vi "Init.vi"(8 "error in (no error)":errorcluster, 11 "reference in":refnum<class "TestView_Base.lvclass">) -> (0 "error out":errorcluster, 3 "reference in":refnum<class "TestView_Base.lvclass">)   [LabVIEW 2022 SP3, in "TestView_Base.lvlib" / "TestView_Base.lvclass"]
uses:
  TestView_Base.lvclass
  Components/ViPER.lvlibp/ViPER.lvclass
  C:/Projects/Medulla/ViPER/Examples/Flux_Capacitor_Tester/Components/ViPER.lvlibp/ViPER.lvclass
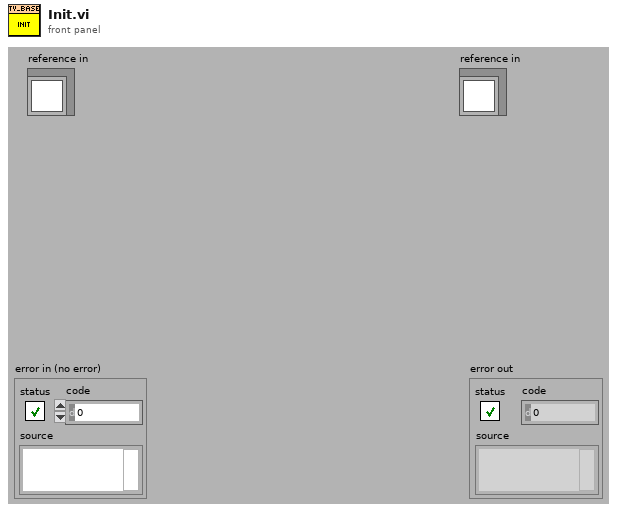
[diagram p1: front panel]
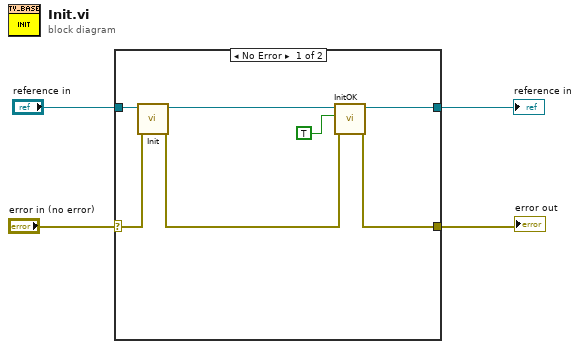
[diagram p0: block diagram]
diagram:
  n1 = case shown="No Error" "error in (no error)" {
    selector: "error in (no error)" -> [w10 w13]
    tunnel: [w8 w13] -> w3
    tunnel: [w9 w12] -> w1
    tunnel: "reference in" -> [w11 w12]
    frame No Error {
      n2 = call-parent "Init.vi"("error in (no error)"=w10, "reference in"=w11) -> ("error out"=w5:errorcluster, "reference out"=w6:refnum<class "TestView_Base.lvclass">)  [unwired: 8 in]
      n3 = call "InitOK.vi"("error in (no error)"=w5, "Init OK?"=TRUE, "reference in"=w6) -> ("error out"=w8:errorcluster, "reference out"=w9:refnum<class "TestView_Base.lvclass">)  [unwired: 7 in]
    }
    frame Error {
    }
  }
  "error out" <- w3
  "reference in" <- w1
